vi "encodeFixedInt.vi"(3 "FixedInt8":i8) -> (1 "Array":u8[](array[numeric]) format="%.0x")   [LabVIEW 2015, in "MsgPack.lvlib"]
uses:
  MsgPack.lvlib
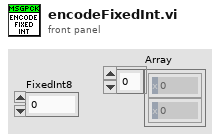
[diagram p1: front panel]
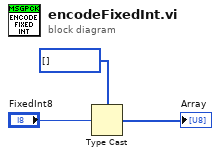
[diagram p0: block diagram]
diagram:
  n1 = Type Cast(type=u8[] [], x="FixedInt8") -> (*(type *) &x=→"Array":u8[])
